vi "Accumulated heat Loss At End.vi"(11 "Proto in":refnum<class "Heat Map.lvclass">) -> (2 "Min Heat":i32, 3 "Proto out":refnum<class "Heat Map.lvclass">)   [LabVIEW 2021, in "Heat Map.lvclass"]
uses:
  Heat Map.lvclass
  Heat Map.lvclass/Heat Map.ctl
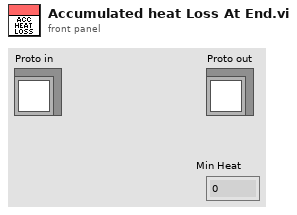
[diagram p1: front panel]
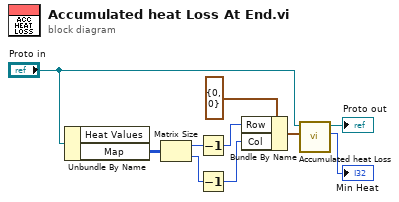
[diagram p0: block diagram]
diagram:
  n1 = Unbundle By Name("Proto in") -> ("Map"=w9:i32[][])  [unwired: 1 out]
  n2 = Matrix Size(0:w9) -> (1:w8:i32, 2:w7:i32)
  n3 = Decrement(x=w8) -> (x-1=w4:i32)
  n4 = Decrement(x=w7) -> (x-1=w3:i32)
  n5 = Bundle By Name(cluster=cluster{"Row":i32, "Col":i32} {"Row"=0, "Col"=0} ("Coord"), "Row"=w4, "Col"=w3) -> (w2:cluster{"Row":i32, "Col":i32})
  n6 = call "Accumulated heat Loss.vi"("Coord"=w2, "Proto in"="Proto in") -> ("Min Heat"=→"Min Heat":i32, "Proto out"=→"Proto out":refnum<class "Heat Map.lvclass">)  [unwired: 8 in]
